vi "Scripting Demo.vi"   [LabVIEW 2024]
uses:
  <vilib>/Utility/miscctls.llb/LVFontTypeDef.ctl
types:
  T1 = typedef "LVFontTypeDef.ctl" = cluster{"Font Name":string, "Size":u16, "Bold":bool, "Italic":bool, "Underline":bool, "Strikeout":bool, "Color":u32}
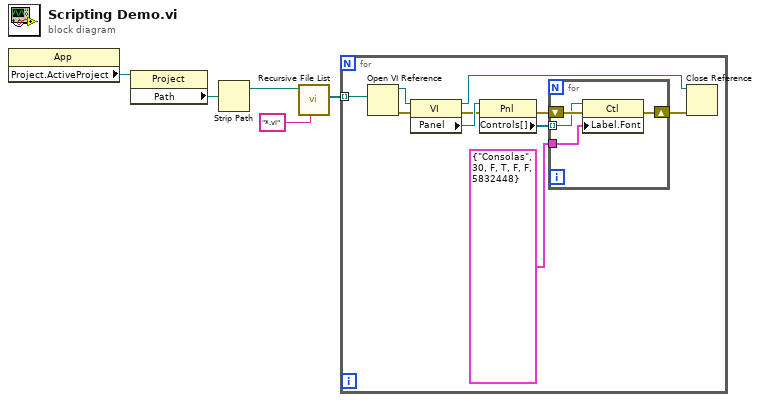
[diagram p0: block diagram]
diagram:
  n1 = property class="App"() -> ("Project.ActiveProject"=w5:refnum<vi>)  [unwired: 2 in, 2 out]
  n2 = property class="Project"(reference=w5) -> ("Path"=w4:path)  [unwired: 1 in, 2 out]
  n3 = Strip Path(path=w4) -> (stripped path=w1:path)  [unwired: 1 out]
  n4 = call <vilib>:"Recursive File List.vi"("pattern"="*.vi", "Folder Path"=w1) -> ("All Files in Dir"=w2:path[])  [unwired: 5 in, 4 out]
  n5 = for {
    tunnel: w2 -> [w6] mode=indexing
    n6 = Open VI Reference(vi path=w6) -> (vi reference=w15:refnum<vi>, error out=w14:errorcluster)  [unwired: 5 in]
    n7 = property class="VI"(reference=w15, error in=w14) -> (reference out=w8:refnum<vi>, error out=w11:errorcluster, "Panel"=w13:refnum<vi>)
    n8 = property class="Pnl"(reference=w13, error in=w11) -> (error out=w10:errorcluster, "Controls[]"=w12:refnum<vi>[])  [unwired: 1 out]
    n9 = for {
      tunnel: w12 -> [w17] mode=indexing
      shift-right: [w18] -> w9
      shift-left: w10 -> [w19]
      tunnel: T1 {"Font Name"="Consolas", "Size"=30, "Bold"=FALSE, "Italic"=TRUE, "Underline"=FALSE, "Strikeout"=FALSE, "Color"=5832448} ("Label.Font") -> [w16]
      n10 = property class="Ctl"(reference=w17, error in=w19, "Label.Font"=w16) -> (error out=w18:errorcluster)  [unwired: 1 out]
    }
    n11 = Close Reference(reference=w8, error in (no error)=w9) -> ()  [unwired: 1 out]
  }
